vi "UI Update Messages.vi"(8 "error in (no error)":errorcluster, 10 "UserMessage":string, 11 "Model_AMC in":refnum<class "Model_AMC.lvclass">) -> (0 "error out":errorcluster, 3 "Model_AMC out":refnum<class "Model_AMC.lvclass">)   [LabVIEW 2021, in "Model_AMC.lvclass"]
uses:
  Model_AMC.lvclass
  Model_AMC.lvclass/Model_AMC.ctl
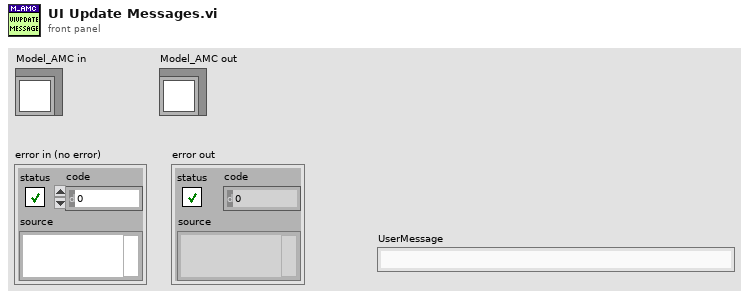
[diagram p1: front panel]
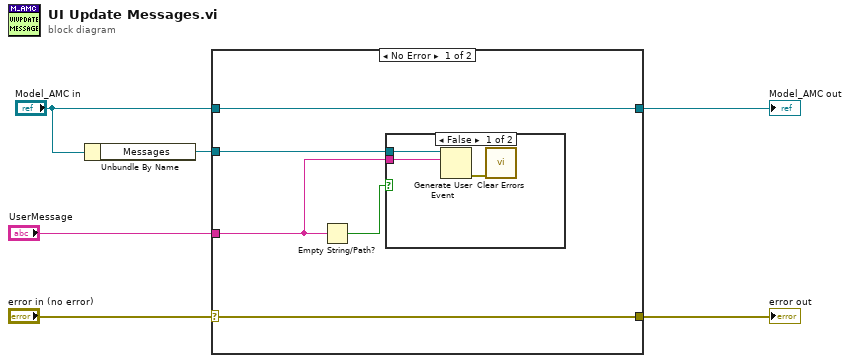
[diagram p0: block diagram]
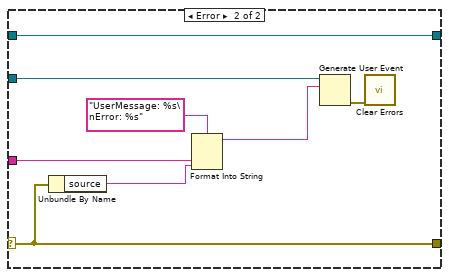
[diagram p3: hidden frame]
diagram:
  n1 = Unbundle By Name("Model_AMC in") -> ("Messages"=w4:refnum<user-event>)
  n2 = case shown="No Error" "error in (no error)" {
    selector: "error in (no error)" -> [w10 w19]
    tunnel: [w10 w19] -> w5
    tunnel: [w11 w22] -> w2
    tunnel: "Model_AMC in" -> [w11 w22]
    tunnel: w4 -> [w9 w20]
    tunnel: "UserMessage" -> [w8 w17]
    frame No Error {
      n3 = Empty String/Path?(string/path=w8) -> (empty?=w7:bool)
      n4 = case shown="False" w7 {
        tunnel: w9 -> [w13 _]
        tunnel: w8 -> [w12 _]
        frame False {
          n5 = Generate User Event(user event=w13, event data cluster=w12) -> (error out=w14:errorcluster)  [unwired: 2 in, 1 out]
          n6 = call <vilib>:"Clear Errors.vi"("error in (no error)"=w14) -> ()  [unwired: 5 in, 2 out]
        }
        frame True {
        }
      }
    }
    frame Error {
      n7 = Unbundle By Name(w19) -> ("source"=w16:string)
      n8 = Format Into String(format string="UserMessage: %s\nError: %s", w17, w16) -> (resulting string=w15:string)  [unwired: 2 in, 1 out]
      n9 = Generate User Event(user event=w20, event data cluster=w15) -> (error out=w21:errorcluster)  [unwired: 2 in, 1 out]
      n10 = call <vilib>:"Clear Errors.vi"("error in (no error)"=w21) -> ()  [unwired: 5 in, 2 out]
    }
  }
  "error out" <- w5
  "Model_AMC out" <- w2
